vi "VI Server_Get TabControl Cluster From Refference w_o Merging.vi"(8 "error in":errorcluster, 9 "Tab Control.Reference":refnum<vi>, 11 "VI Server Cluster":T1) -> (0 "error out":errorcluster, 2 "Tab Data Cluster":T1={"Labels"=["Label", "Size", "Font", "Heght", "Width", "Ledding Denominator", "Ledding Nominator", "Label Number", "Microstep Resolution", "X", "Y", "Z", "Italic?", "Underlined?"], "Refs"=[], "VI Ref"=refnum}, 3 "VI Server Cluster.DUP":T1)   [LabVIEW 2020, in "VI Server Toolkit LV2013.lvlib"]
doc: "Retrieves control labels and references of a tab control (reference input) and outputs separate VI server Cluster."
uses:
  VI Server Toolkit LV2013.lvlib
  VI Server_TypeDefs/VI Server_RefsCluster.ctl
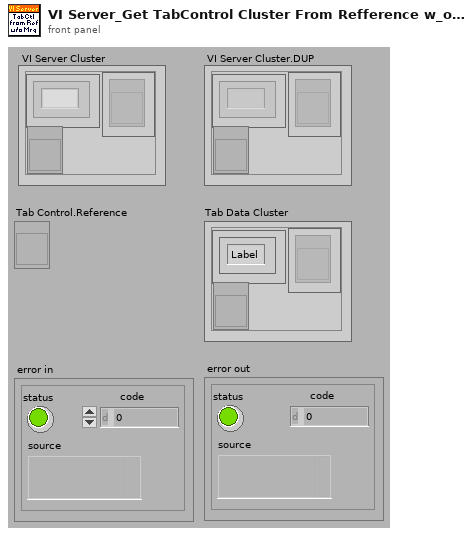
[diagram p1: front panel]
types:
  T1 = typedef "VI Server_RefsCluster.ctl" = cluster{"Labels":string[], "Refs":refnum<vi>[], "VI Ref":refnum<vi>}
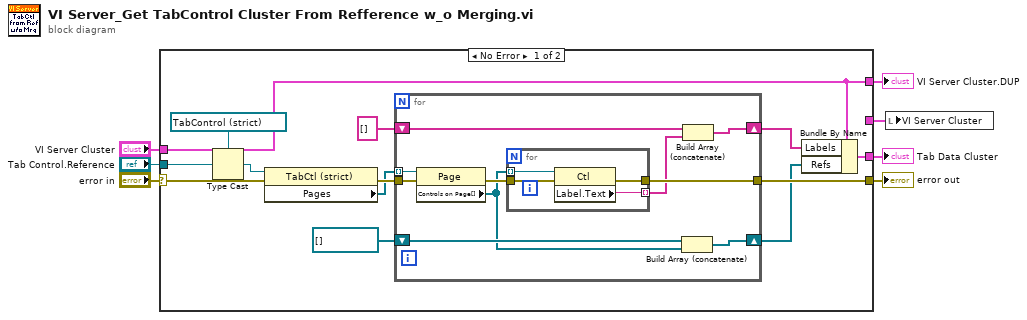
[diagram p0: block diagram]
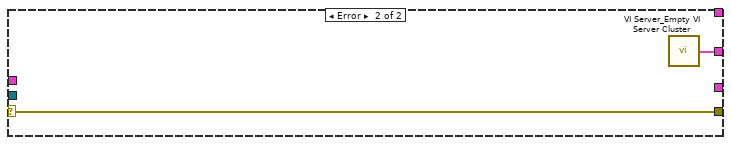
[diagram p2: hidden frame]
diagram:
  n1 = case shown="No Error" "error in" {
    selector: "error in" -> [w14 w36]
    tunnel: "VI Server Cluster" -> [w11 _]
    tunnel: [w20 w36] -> w6
    tunnel: [w15 _] -> w2
    tunnel: "Tab Control.Reference" -> [w13 _]
    tunnel: [w11 _] -> w3
    tunnel: [_ w35] -> w1
    frame No Error {
      n2 = Type Cast(type=refnum<vi> refnum ("Tab Control Ref"), x=w13) -> (*(type *) &x=w12:refnum<vi>)
      n3 = property class="TabCtl (strict)"(reference=w12, error in=w14) -> (error out=w19:errorcluster, "Pages"=w18:refnum<vi>[])  [unwired: 1 out]
      n4 = for {
        tunnel: w19 -> [w29]
        tunnel: [w27] -> w20
        tunnel: w18 -> [w30] mode=indexing
        shift-right: [w24] -> w10
        shift-left: string[] [] -> [w26]
        shift-right: [w22] -> w9
        shift-left: refnum<vi>[] [] ("Controls on Page[]") -> [w23]
        n5 = property class="Page"(reference=w30, error in=w29) -> (error out=w28:errorcluster, "Controls on Page[]"=w21:refnum<vi>[])  [unwired: 1 out]
        n6 = for {
          tunnel: w28 -> [w34]
          tunnel: w21 -> [w33] mode=indexing
          tunnel: [w32] -> w27
          tunnel: [w31] -> w25 mode=indexing
          n7 = property class="Ctl"(reference=w33, error in=w34) -> (error out=w32:errorcluster, "Label.Text"=w31:string)  [unwired: 1 out]
        }
        n8 = Build Array (concatenate)(w23, w21) -> (w22:refnum<vi>[])
        n9 = Build Array (concatenate)(w26, w25) -> (w24:string[])
      }
      n10 = Bundle By Name(cluster=w11, "Labels"=w10, "Refs"=w9) -> (w15:T1)
    }
    frame Error {
      n11 = call "VI Server_Empty VI Server Cluster.vi"() -> ("VI Server Cluster"=w35:T1)  [unwired: 7 in]
    }
  }
  "error out" <- w6
  "VI Server Cluster.DUP" <- w3
  "Tab Data Cluster" <- w2
  n12 = local write "VI Server Cluster"(w1) -> ()
